vi "IN-READ (subvi).vi"(8 "error in (no error)":errorcluster, 11 "ARRAY IN":string[](array[string])) -> (0 "error out":errorcluster, 2 "Entradas":bool[](array[boolean]))   [LabVIEW 2014, in "CAP-USB.lvlib"]
doc: "Detecta el valor de las entradas enviado\npor el CAP-USB"
uses:
  CAP-USB.lvlib
  0-Nivel/Enum DI-Reader.ctl
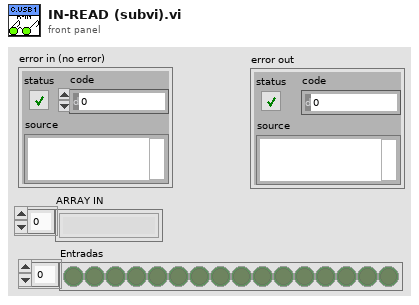
[diagram p1: front panel]
types:
  T1 = typedef "CAP-USB.lvlib/Enum DI-Reader.ctl" = enum16{"IDLE", "Detect XX", "Detect YY", "Valor", ""}
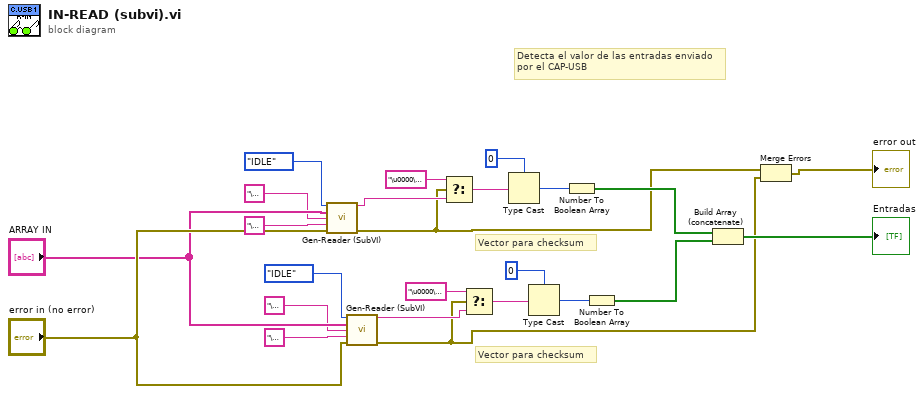
[diagram p0: block diagram]
diagram:
  # "Detecta el valor de las entradas enviado\npor el CAP-USB"
  # "Vector para checksum"
  # "Vector para checksum"
  n1 = call "Gen-Reader (SubVI).vi"("Enum"=Enum_DI-Reader."IDLE", "ARRAY IN"="ARRAY IN", "XX"="\u0003", "YY"="\u0000", "error in (no error)"="error in (no error)") -> ("read buffer"=w13:string, "error out"=w2:errorcluster)  [unwired: 8 in, 1 out]
  n2 = call "Gen-Reader (SubVI).vi"("Enum"=Enum_DI-Reader."IDLE", "ARRAY IN"="ARRAY IN", "XX"="\u0003", "YY"="\u0004", "error in (no error)"="error in (no error)") -> ("read buffer"=w11:string, "error out"=w3:errorcluster)  [unwired: 8 in, 1 out]
  n3 = Select(t="\u0000\u0000", s=w2, f=w13) -> (s? t:f=w19:string)
  n4 = Select(t="\u0000\u0000", s=w3, f=w11) -> (s? t:f=w9:string)
  n5 = Type Cast(type=u8 0 ("default (0 U32)"), x=w19) -> (*(type *) &x=w18:u8)
  n6 = Type Cast(type=u8 0 ("default (0 U32)"), x=w9) -> (*(type *) &x=w8:u8)
  n7 = Number To Boolean Array(number=w18) -> (Boolean array=w23:bool[])
  n8 = Number To Boolean Array(number=w8) -> (Boolean array=w22:bool[])
  n9 = Build Array (concatenate)(w23, w22) -> (→"Entradas":bool[])
  n10 = Merge Errors(w2, w3) -> (→"error out":errorcluster)
